vi "Proportional Correction.vi"(11 "Correction Factor K":dbl) -> ()   [LabVIEW 2017]
uses:
  Globals.vi
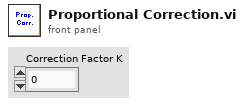
[diagram p1: front panel]
types:
  T1 = cluster{"x shift":dbl, "y shift":dbl, "z shift":dbl, "Theta x":dbl, "Theta y":dbl}
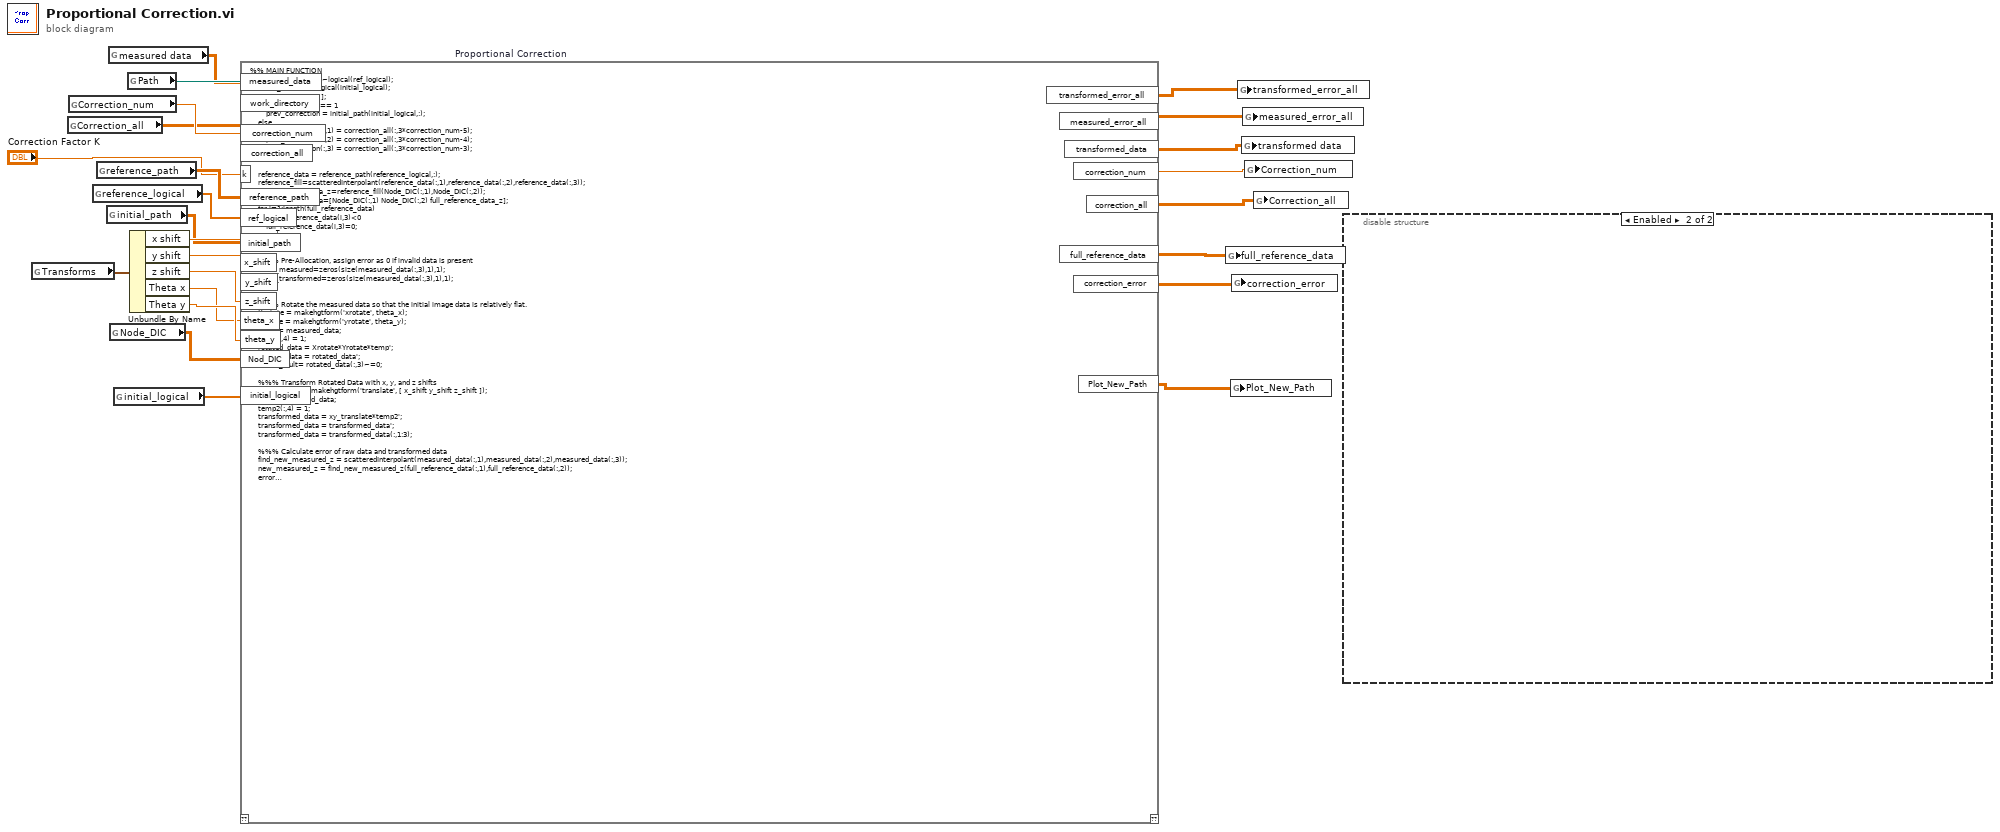
[diagram p0: block diagram]
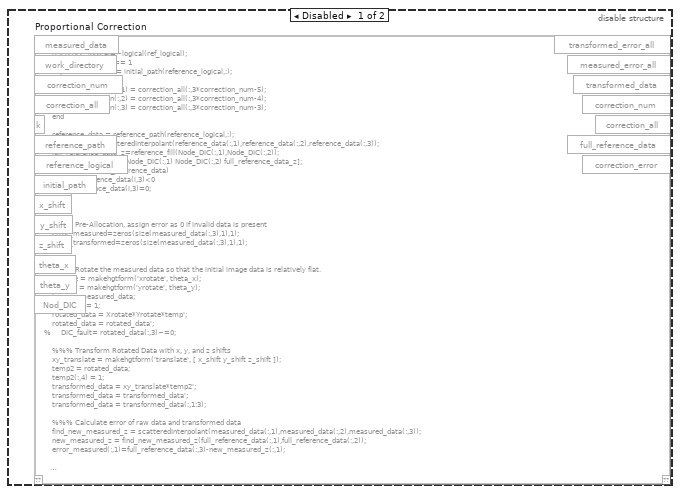
[diagram p2: hidden frame]
diagram:
  n1 = global read "Globals.vi" "Transforms"() -> (w9:T1)
  n2 = global read "Globals.vi" "Correction_all"() -> (w16:dbl[][])
  n3 = global read "Globals.vi" "Correction_num"() -> (w17:dbl)
  n4 = global read "Globals.vi" "reference_logical"() -> (w7:dbl[])
  n5 = global read "Globals.vi" "reference_path"() -> (w6:dbl[][])
  n6 = global read "Globals.vi" "initial_path"() -> (w8:dbl[][])
  n7 = global read "Globals.vi" "measured data"() -> (w3:dbl[][])
  n8 = global read "Globals.vi" "Node_DIC"() -> (w15:dbl[][])
  n9 = global read "Globals.vi" "initial_logical"() -> (w1:dbl[])
  n10 = global read "Globals.vi" "Path"() -> (w4:path)
  n11 = Unbundle By Name(w9) -> ("x shift"=w10:dbl, "y shift"=w11:dbl, "z shift"=w12:dbl, "Theta x"=w13:dbl, "Theta y"=w14:dbl)
  n12 = script code="%% MAIN FUNCTION\n    reference_logical=~logical(ref_logical); \n    initial_logical=~logical(initial_logical);\n    prev_correction=[];\n    if correction_num == 1\n        prev_correction = initial_path(initial_logical,:);\n    else\n        prev_correction(:,1) = correction_all(:,3*correction_num-5);\n        prev_correction(:,2) = correction_all(:,3*correction_num-4);\n        prev_correction(:,3) = correction_all(:,3*correction_num-3);\n    end\n\n    reference_data = reference_path(reference_logical,:);\n    reference_fill=scatteredInterpolant(reference_data(:,1),reference_data(:,2),reference_data(:,3));\n    full_reference_data_z=reference_fill(Node_DIC(:,1),Node_DIC(:,2));\n    full_reference_data=[Node_DIC(:,1) Node_DIC(:,2) full_reference_data_z];\n    for i=1:length(full_reference_data)\n        if full_reference_data(i,3)<0\n        full_reference_data(i,3)=0;\n        end\n    end\n\n    %%% Pre-Allocation, assign error as 0 if invalid data is present\n    error_measured=zeros(size(measured_data(:,3),1),1);\n    error_transformed=zeros(size(measured_data(:,3),1),1);\n\n    \n    %%% Rotate the measured data so that the initial image data is relatively flat.\n    Xrotate = makehgtform('xrotate', theta_x);\n    Yrotate = makehgtform('yrotate', theta_y);\n    temp = measured_data;\n    temp(:,4) = 1;\n    rotated_data = Xrotate*Yrotate*temp';\n    rotated_data = rotated_data';\n%     DIC_fault= rotated_data(:,3)~=0;\n    \n    %%% Transform Rotated Data with x, y, and z shifts\n    xy_translate = makehgtform('translate', [ x_shift y_shift z_shift ]);\n    temp2 = rotated_data;\n    temp2(:,4) = 1;\n    transformed_data = xy_translate*temp2';\n    transformed_data = transformed_data';\n    transformed_data = transformed_data(:,1:3);\n    \n    %%% Calculate error of raw data and transformed data\n    find_new_measured_z = scatteredInterpolant(measured_data(:,1),measured_data(:,2),measured_data(:,3));\n    new_measured_z = find_new_measured_z(full_reference_data(:,1),full_reference_data(:,2));\n    error_measured(:,1)=full_reference_data(:,3)-new_measured_z(:,1);\n    \n    find_new_transformed_z = scatteredInterpolant(transformed_data(:,1),transformed_data(:,2),transformed_data(:,3));\n    new_transformed_z = find_new_transformed_z(full_reference_data(:,1),full_reference_data(:,2));\n    error_transformed(:,1)=full_reference_data(:,3)-new_transformed_z(:,1);\n    \n    transformed_data(:,1:2) = full_reference_data(:,1:2);\n    transformed_data(:,3) = new_transformed_z(:,1);\n\n    %_____________________________________________________________________________________________________________________\n%     figure(7)\n% %     plot3(reference_data(:,1),reference_data(:,2),reference_data(:,3))\n%     plot3(full_reference_data(:,1),full_reference_data(:,2),full_reference_data(:,3),'r')\n%     hold on\n%     plot3(transformed_data(:,1),transformed_data(:,2),transformed_data(:,3),'k')\n%     hold off\n%     figure(8)\n%     plot3(transformed_data(:,1),transformed_data(:,2),transformed_data(:,3),'b')\n    %_____________________________________________________________________________________________________________________\n    \n    find_correction_error=scatteredInterpolant(full_reference_data(:,1),full_reference_data(:,2),error_transformed(:,1));\n    correction_error=find_correction_error(reference_data(:,1),reference_data(:,2));\n    \n    find_previous_path=scatteredInterpolant(prev_correction(:,1),prev_correction(:,2),prev_correction(:,3));\n    prev_correction=[];\n    prev_correction(:,1:2)=reference_data(:,1:2);\n    prev_correction(:,3)=find_previous_path(reference_data(:,1),reference_data(:,2));\n    \n    %%% CORRECTION CALCULATION\n        %%% Assign New Correction\n        current_correction=[];\n        current_correction(:,1:2)=reference_data(:,1:2);\n\n        current_correction(:,3)=prev_correction(:,3)+k*correction_error;\n        % If current correction is negative, set to 0 (cannot negatively form)\n        for i = 1:length(current_correction)\n            if current_correction(i,3) < 0 \n                current_correction(i,3) = 0;\n            end\n        end\n            \n        %%% Assign as New Correction on Correction Array\n           correction_all(:,3*correction_num-2) = current_correction(:,1);\n           correction_all(:,3*correction_num-1) = current_correction(:,2);\n           correction_all(:,3*correction_num) = current_correction(:,3);\n\n     %%% PLOT NEW PATH\n        points=zeros(length(current_correction),3);\n        for i=1:length(current_correction)\n            points(i,1)=current_correction(i,1);\n            points(i,2)=current_correction(i,2);\n            points(i,3)=current_correction(i,3);\n            points(i,4)=1;\n        end\n        Plot_New_Path=[0];\n        Plot_New_Path = points;\n        \n%         plot3(Plot_New_Path(:,1),Plot_New_Path(:,2),Plot_New_Path(:,3),'k');\n%         hold on;\n%         scatter3(Plot_New_Path(:,1),Plot_New_Path(:,2),Plot_New_Path(:,3),'r');\n%         hold off;\n        \n        %%% Store error in matrix to reference after multiple corrections\n        measured_error_all(:,correction_num) = error_measured;\n        transformed_error_all(:,correction_num) = error_transformed;" "Proportional Correction"("measured_data"=w3, "work_directory"=w4, "correction_num"=w17, "correction_all"=w16, "k"="Correction Factor K", "reference_path"=w6, "ref_logical"=w7, "initial_path"=w8, "theta_x"=w13, "theta_y"=w14, "x_shift"=w10, "y_shift"=w11, "z_shift"=w12, "Nod_DIC"=w15, "initial_logical"=w1) -> ("transformed_error_all"=w20:dbl[][], "measured_error_all"=w21:dbl[][], "transformed_data"=w22:dbl[][], "correction_num"=w19:dbl, "correction_all"=w18:dbl[][], "full_reference_data"=w23:dbl[][], "correction_error"=w24:dbl[][], "Plot_New_Path"=w2:dbl[][])  [unwired: 1 in, 1 out]
  n13 = global write "Globals.vi" "full_reference_data"(w23) -> ()
  n14 = global write "Globals.vi" "Plot_New_Path"(w2) -> ()
  n15 = global write "Globals.vi" "correction_error"(w24) -> ()
  n16 = global write "Globals.vi" "transformed_error_all"(w20) -> ()
  n17 = global write "Globals.vi" "transformed data"(w22) -> ()
  n18 = global write "Globals.vi" "measured_error_all"(w21) -> ()
  n19 = global write "Globals.vi" "Correction_num"(w19) -> ()
  n20 = global write "Globals.vi" "Correction_all"(w18) -> ()
  n21 = disable-structure shown="Enabled" {
    frame Disabled {
      n22 = script code="%% MAIN FUNCTION\n    reference_logical=~logical(ref_logical); \n    if correction_num == 1\n        prev_correction = initial_path(reference_logical,:);\n    else\n        prev_correction(:,1) = correction_all(:,3*correction_num-5);\n        prev_correction(:,2) = correction_all(:,3*correction_num-4);\n        prev_correction(:,3) = correction_all(:,3*correction_num-3);\n    end\n\n    reference_data = reference_path(reference_logical,:);\n    reference_fill=scatteredInterpolant(reference_data(:,1),reference_data(:,2),reference_data(:,3));\n    full_reference_data_z=reference_fill(Node_DIC(:,1),Node_DIC(:,2));\n    full_reference_data=[Node_DIC(:,1) Node_DIC(:,2) full_reference_data_z];\n    for i=1:length(full_reference_data)\n        if full_reference_data(i,3)<0\n        full_reference_data(i,3)=0;\n        end\n    end\n\n    %%% Pre-Allocation, assign error as 0 if invalid data is present\n    error_measured=zeros(size(measured_data(:,3),1),1);\n    error_transformed=zeros(size(measured_data(:,3),1),1);\n\n    \n    %%% Rotate the measured data so that the initial image data is relatively flat.\n    Xrotate = makehgtform('xrotate', theta_x);\n    Yrotate = makehgtform('yrotate', theta_y);\n    temp = measured_data;\n    temp(:,4) = 1;\n    rotated_data = Xrotate*Yrotate*temp';\n    rotated_data = rotated_data';\n%     DIC_fault= rotated_data(:,3)~=0;\n    \n    %%% Transform Rotated Data with x, y, and z shifts\n    xy_translate = makehgtform('translate', [ x_shift y_shift z_shift ]);\n    temp2 = rotated_data;\n    temp2(:,4) = 1;\n    transformed_data = xy_translate*temp2';\n    transformed_data = transformed_data';\n    transformed_data = transformed_data(:,1:3);\n    \n    %%% Calculate error of raw data and transformed data\n    find_new_measured_z = scatteredInterpolant(measured_data(:,1),measured_data(:,2),measured_data(:,3));\n    new_measured_z = find_new_measured_z(full_reference_data(:,1),full_reference_data(:,2));\n    error_measured(:,1)=full_reference_data(:,3)-new_measured_z(:,1);\n    \n    find_new_transformed_z = scatteredInterpolant(transformed_data(:,1),transformed_data(:,2),transformed_data(:,3));\n    new_transformed_z = find_new_transformed_z(full_reference_data(:,1),full_reference_data(:,2));\n    error_transformed(:,1)=full_reference_data(:,3)-new_transformed_z(:,1);\n    \n    transformed_data(:,1:2) = full_reference_data(:,1:2);\n    transformed_data(:,3) = new_transformed_z(:,1);\n\n    %_____________________________________________________________________________________________________________________\n    figure(7)\n%     plot3(reference_data(:,1),reference_data(:,2),reference_data(:,3))\n    plot3(full_reference_data(:,1),full_reference_data(:,2),full_reference_data(:,3),'r')\n    hold on\n    plot3(transformed_data(:,1),transformed_data(:,2),transformed_data(:,3),'k')\n    hold off\n    figure(8)\n    plot3(transformed_data(:,1),transformed_data(:,2),transformed_data(:,3),'b')\n    %_____________________________________________________________________________________________________________________\n    \n    find_correction_error=scatteredInterpolant(full_reference_data(:,1),full_reference_data(:,2),error_transformed(:,1));\n    correction_error=find_correction_error(reference_data(:,1),reference_data(:,2));\n    \n    \n    %%% CORRECTION CALCULATION\n        %%% Assign New Correction\n        current_correction(:,1:2)=reference_data(:,1:2);\n        current_correction(:,3)=prev_correction(:,3)+k*correction_error;\n\n        % If current correction is negative, set to 0 (cannot negatively form)\n        for i = 1:length(current_correction)\n            if current_correction(i,3) < 0 \n                current_correction(i,3) = 0;\n            end\n        end\n            \n        %%% Assign as New Correction on Correction Array\n           correction_all(:,3*correction_num-2) = current_correction(:,1);\n           correction_all(:,3*correction_num-1) = current_correction(:,2);\n           correction_all(:,3*correction_num) = current_correction(:,3);\n\n     %%% PLOT NEW PATH\n        points=zeros(length(current_correction),3);\n        for i=1:length(current_correction)\n            points(i,1)=current_correction(i,1);\n            points(i,2)=current_correction(i,2);\n            points(i,3)=current_correction(i,3);\n            points(i,4)=1;\n        end\n        Xrotate=makehgtform('xrotate',(pi/2));\n        Plot_New_Path = points;\n        Plot_New_Path = Xrotate*Plot_New_Path';\n        Plot_New_Path = Plot_New_Path';\n        \n        plot3(Plot_New_Path(:,1),Plot_New_Path(:,2),Plot_New_Path(:,3),'k');\n        hold on;\n        scatter3(Plot_New_Path(:,1),Plot_New_Path(:,2),Plot_New_Path(:,3),'r');\n        hold off;\n        \n        %%% Store error in matrix to reference after multiple corrections\n        measured_error_all(:,correction_num) = error_measured;\n        transformed_error_all(:,correction_num) = error_transformed;" "Proportional Correction"() -> ()  [unwired: 15 in, 8 out]
    }
    frame Enabled {
    }
  }
